vi "Calc - WBcor.vi"(10 "WBMeas":dbl, 11 "dPAMB":dbl) -> (3 "WBCor":dbl)   [LabVIEW 2018, in "Controller (Host).lvlib"]
uses:
  Controller (Host).lvlib
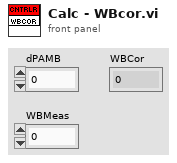
[diagram p1: front panel]
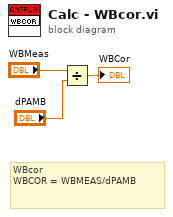
[diagram p0: block diagram]
diagram:
  # "WBcor \nWBCOR = WBMEAS/dPAMB"
  n1 = Divide(x="WBMeas", y="dPAMB") -> (x/y=→"WBCor":dbl)
